vi "RFSG Change Signal.vi"(7 "Initial RFSG Reference":refnum<k15>, 8 "error in (no error)":errorcluster, 10 "Samples Per Cycle":i32, 11 "RFSG Reference In":refnum<k15>) -> (0 "error out":errorcluster, 3 "RFSG Reference Out":refnum<k15>)   [LabVIEW 2021]
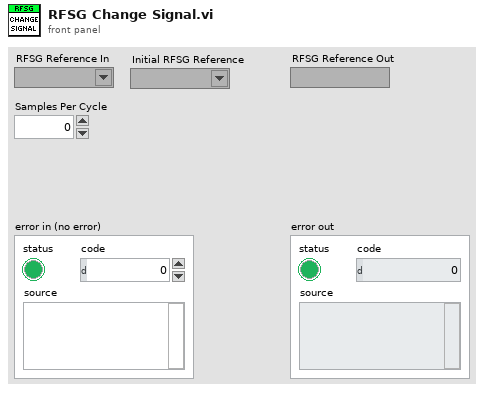
[diagram p1: front panel]
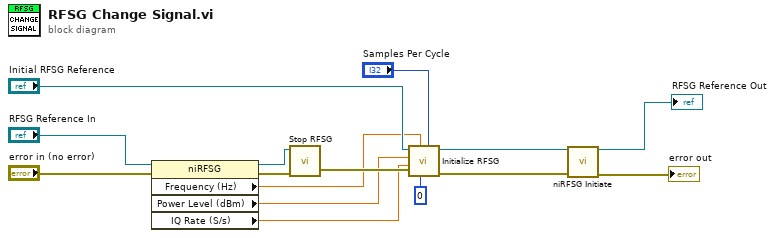
[diagram p0: block diagram]
diagram:
  n1 = property class="niRFSG"(reference="RFSG Reference In", error in="error in (no error)") -> (reference out=w4:refnum<k15>, error out=w12:errorcluster, "Frequency (Hz)"=w6:dbl, "Power Level (dBm)"=w7:dbl, "IQ Rate (S/s)"=w8:dbl)
  n2 = call "Stop RFSG.vi"("error in (no error)"=w12, "RFSG Reference In"=w4) -> ("error out"=w11:errorcluster)  [unwired: 9 in]
  n3 = call "Initialize RFSG.vi"("Frequency Offset"="Samples Per Cycle", "Selected Waveform"=u16 0, "Center Frequency"=w6, "error in (no error)"=w11, "IQ Rate"=w8, "Power Level"=w7, "RFSG Reference In"="Initial RFSG Reference") -> ("error out"=w3:errorcluster, "RFSG Reference Out"=w2:refnum<k15>)  [unwired: 1 in, 2 out]
  n4 = call <instrlib>:"niRFSG Initiate.vi"("instrument handle"=w2, "error in"=w3) -> ("instrument handle out"=→"RFSG Reference Out":refnum<k15>, "error out"=→"error out":errorcluster)  [unwired: 12 in]
